vi "Events.vi"() -> ()   [LabVIEW 2018]
uses:
  Spels.AutomationTools.RemoteFunctionalControlService.dll
panel:
  in  "Set Inputs Enabled":bool
  in  "Reset":bool
  in  "Do FC":bool
  out "FPGA OE":bool
  in  "stop":bool
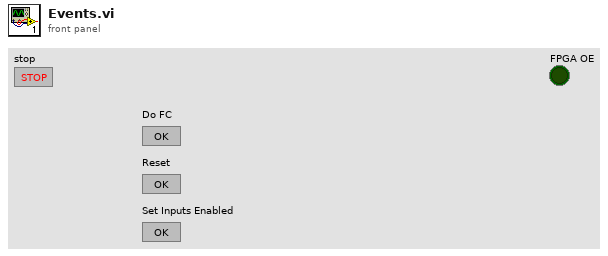
[diagram p1: front panel]
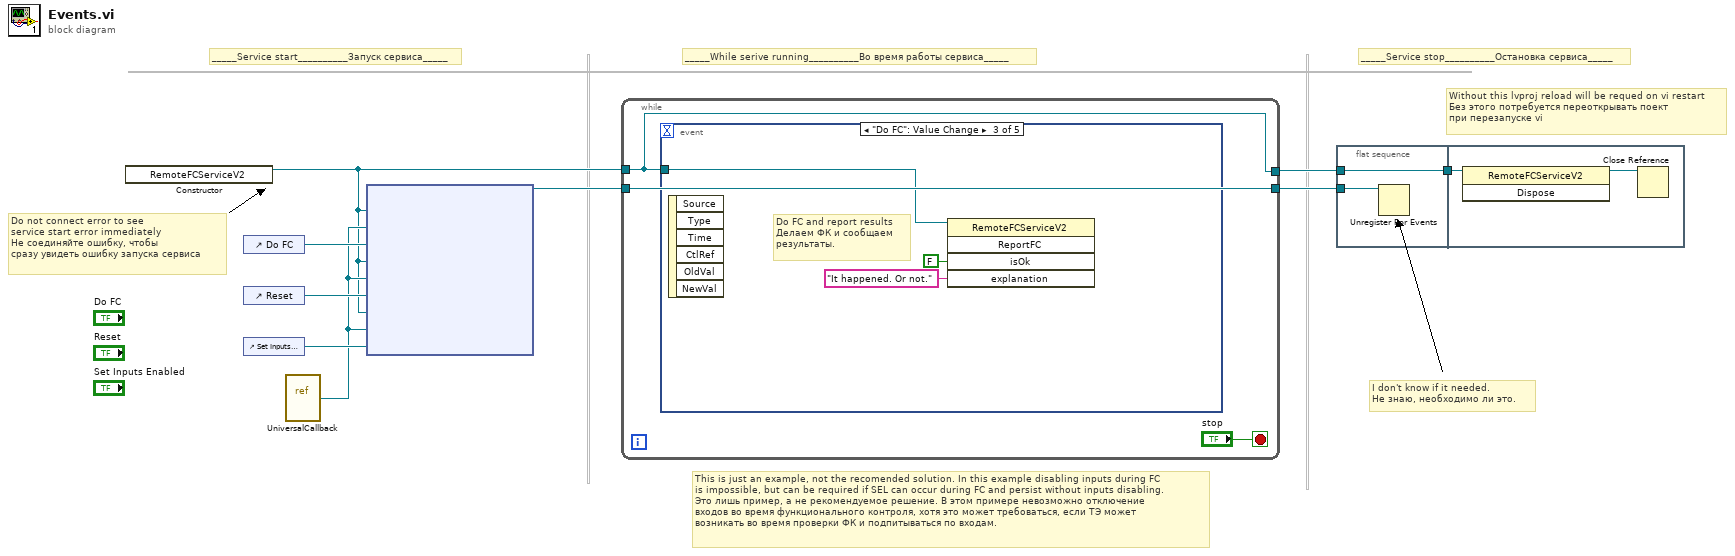
[diagram p0: block diagram]
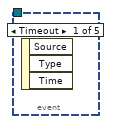
[diagram p2: hidden frame]
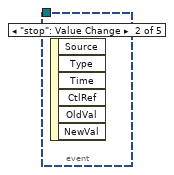
[diagram p3: hidden frame]
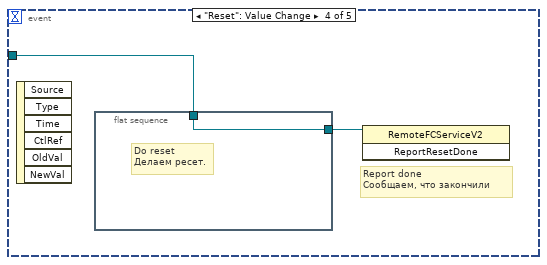
[diagram p4: hidden frame]
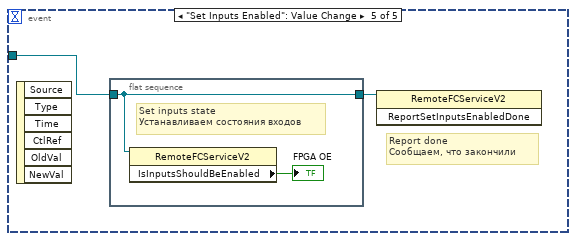
[diagram p5: hidden frame]
diagram:
  # "I don't know if it needed.\nНе знаю, необходимо ли это."
  # "This is just an example, not the recomended solution. In this example disabling inputs during FC\nis impossible, but can be required if SEL can occur during FC and persist without inputs disabling.\nЭто лишь пример, а не рекомендуемое решение. В этом примере невозможно отключение \nвходов во время функционального контроля, хотя это может требоваться, если ТЭ может\nвозникать во время проверки ФК и подпитываться по входам."
  # "Do not connect error to see \nservice start error immediately\nНе соединяйте ошибку, чтобы \nсразу увидеть ошибку запуска сервиса"
  # "Without this lvproj reload will be requed on vi restart\nБез этого потребуется переоткрывать поект \nпри перезапуске vi"
  # "_____Service stop__________Остановка сервиса_____"
  # "_____While serive running__________Во время работы сервиса_____"
  # "_____Service start__________Запуск сервиса_____"
  n1 = constructor class="RemoteFCServiceV2"() -> (reference out=w4:refnum<k24>)  [unwired: 3 in, 2 out]
  n2 = control-ref of="Do FC"() -> (w7:refnum<vi>)
  n3 = control-ref of="Reset"() -> (w8:refnum<vi>)
  n4 = control-ref of="Set Inputs Enabled"() -> (w9:refnum<vi>)
  n5 = vi-ref "UniversalCallback.vi"() -> ("vi reference"=w6:refnum<vi>)
  n6 = node(w4, w6, w7, w4, w6, w8, w4, w6, w9) -> (w3:refnum<k27>)  [unwired: 2 in, 1 out]
  n7 = while {
    tunnel: w4 -> [w11]
    tunnel: [w11] -> w5
    tunnel: w3 -> [w10]
    tunnel: [w10] -> w1
    stop <- "stop" stop-if-true
    n8 = event shown="[2] \"Do FC\": Value Change" {
      selector: _ -> [_ _ _ _ _]
      dyn-events: _ -> [_ _ _ _ _]
      timeout: _ -> [_ _ _ _ _]
      tunnel: w11 -> [_ _ w13 w16 w19]
      event Timeout {
        n9 = event-data() -> ()  [unwired: 1 in, 3 out]
      }
      event "stop": Value Change {
        n10 = event-data() -> ()  [unwired: 1 in, 6 out]
      }
      event "Do FC": Value Change {
        # "Do FC and report results\nДелаем ФК и сообщаем\nрезультаты."
        n11 = event-data() -> ()  [unwired: 1 in, 6 out]
        n12 = invoke class="RemoteFCServiceV2" method="ReportFC"(reference=w13, "isOk"=FALSE, "explanation"="It happened. Or not.") -> ()  [unwired: 2 in, 5 out]
      }
      event "Reset": Value Change {
        # "Report done\nСообщаем, что закончили"
        n13 = event-data() -> ()  [unwired: 1 in, 6 out]
        n14 = flat-sequence {
          tunnel: [w18] -> w17
          tunnel: w16 -> [w18]
          frame #0 {
            # "Do reset\nДелаем ресет."
          }
        }
        n15 = invoke class="RemoteFCServiceV2" method="ReportResetDone"(reference=w17) -> ()  [unwired: 2 in, 3 out]
      }
      event "Set Inputs Enabled": Value Change {
        # "Report done\nСообщаем, что закончили"
        n16 = event-data() -> ()  [unwired: 1 in, 6 out]
        n17 = flat-sequence {
          tunnel: w19 -> [w21]
          tunnel: [w21] -> w20
          frame #0 {
            # "Set inputs state\nУстанавливаем состояния входов"
            n18 = property class="RemoteFCServiceV2"(reference=w21) -> ("IsInputsShouldBeEnabled"=→"FPGA OE":bool)  [unwired: 1 in, 2 out]
          }
        }
        n19 = invoke class="RemoteFCServiceV2" method="ReportSetInputsEnabledDone"(reference=w20) -> ()  [unwired: 2 in, 3 out]
      }
    }
  }
  n20 = flat-sequence {
    tunnel: w5 -> [w24]
    tunnel: [w24] -> w2
    tunnel: w1 -> [w23]
    tunnel: w2 -> [w25]
    frame #0 {
      n21 = Unregister For Events(event registration refnum=w23) -> ()  [unwired: 1 in, 1 out]
    }
    frame #1 {
      n22 = invoke class="RemoteFCServiceV2" method="Dispose"(reference=w25) -> (reference out=w26:refnum<k24>)  [unwired: 2 in, 2 out]
      n23 = Close Reference(reference=w26) -> ()  [unwired: 1 in, 1 out]
    }
  }
